vi "Write remote port.vi"(8 "error in (no error)":errorcluster, 10 "remote port":u16=6341, 11 "Client Config in":refnum<class "Client Config.lvclass">) -> (0 "error out":errorcluster, 3 "Client Config out":refnum<class "Client Config.lvclass">)   [LabVIEW 2016, in "Client Controller.lvlib" / "Client Config.lvclass"]
uses:
  Client Config.lvclass
  Client Config.lvclass/Client Config.ctl
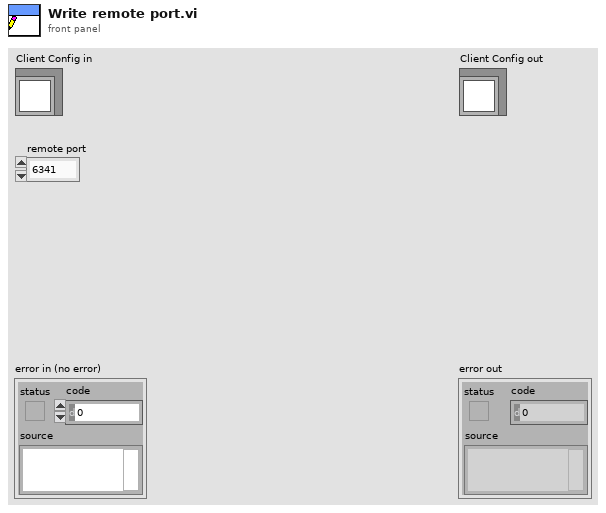
[diagram p1: front panel]
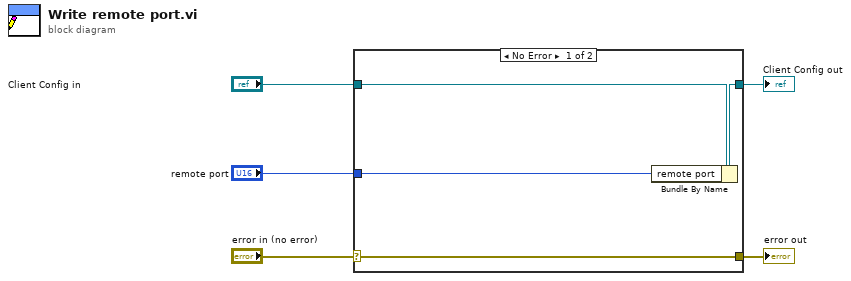
[diagram p0: block diagram]
diagram:
  n1 = case shown="No Error" "error in (no error)" {
    selector: "error in (no error)" -> [w9 w10]
    tunnel: [w9 w10] -> w4
    tunnel: [w7 w11] -> w2
    tunnel: "Client Config in" -> [w8 w11]
    tunnel: "remote port" -> [w6 _]
    frame No Error {
      n2 = Bundle By Name(cluster=w8, "remote port"=w6) -> (w7:refnum<class "Client Config.lvclass">)
    }
    frame Error {
    }
  }
  "error out" <- w4
  "Client Config out" <- w2
